vi "836_Safe Image Get Image.vi"(6 "Video Mode":i32, 8 "error in":errorcluster, 9 "Operation":T3(ring), 10 "Image In":T1, 11 "Session In":T2) -> (0 "error out":errorcluster, 1 "Image Data String":string, 2 "Image Out":T1, 3 "Session Out":T2)   [LabVIEW 2015]
uses:
  <vilib>/userdefined/High Color/IMAQdx.ctl
  <vilib>/vision/Image Controls.llb/IMAQ Image.ctl
  <vilib>/vision/driver/IMAQdx.llb/IMAQdx Buffer Number Mode.ctl
  <resource>/objmgr/imaqdx.rc
  <vilib>/vision/driver/NI_Vision_Acquisition_Software.lvlib
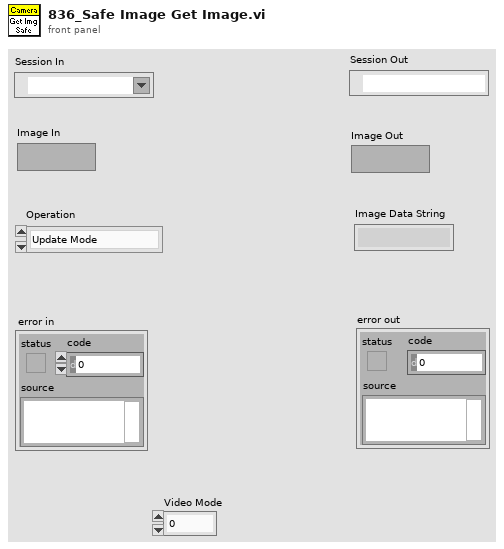
[diagram p1: front panel]
types:
  T1 = typedef "IMAQ Image.ctl" = refnum<image>
  T2 = typedef "IMAQdx.ctl" = refnum<k21>
  T3 = enum16{"Update Mode", "Get Image", "Get Image Data"}
  T4 = typedef "NI_Vision_Acquisition_Software.lvlib/IMAQdx Buffer Number Mode.ctl" = enum32{"Next", "Last", "Buffer Number", "Every", "Last New"}
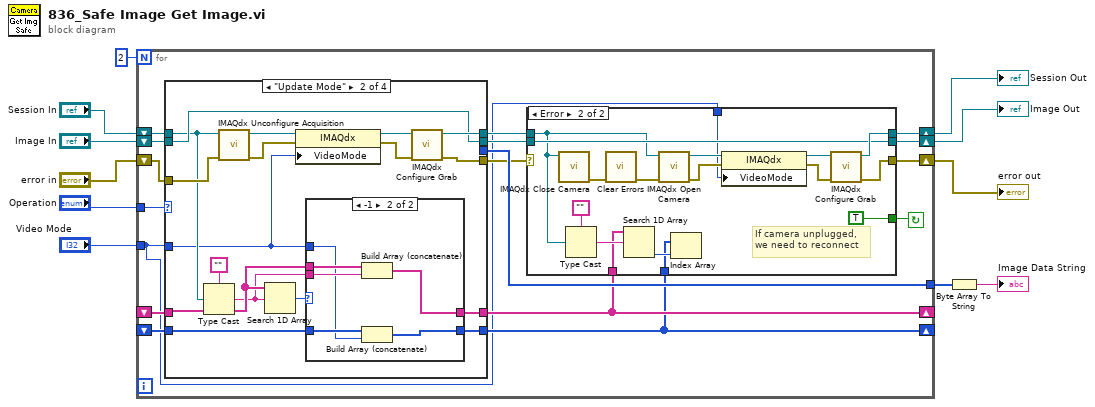
[diagram p0: block diagram]
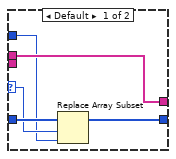
[diagram p4: hidden frame]
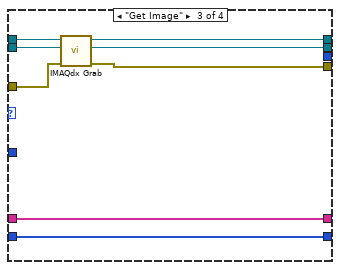
[diagram p5: hidden frame]
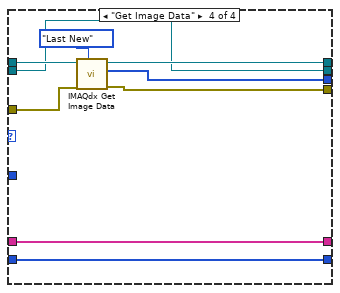
[diagram p6: hidden frame]
diagram:
  n1 = for {
    N: 2 -> [_]
    tunnel: "Operation" -> [w28]
    tunnel: "Video Mode" -> [w12]
    tunnel: [w24] -> w7
    shift-right: [w18] -> w3
    shift-left: "Session In" -> [w27]
    shift-right: [w20] -> w4
    shift-left: "Image In" -> [w26]
    shift-right: [w22] -> w5
    shift-left: "error in" -> [w25]
    shift-right: [w14] -> _
    shift-left: _ -> [w16]
    shift-right: [w13] -> _
    shift-left: _ -> [w15]
    stop <- w17 continue-if-true
    n2 = case shown="\"Update Mode\"" w28 {
      tunnel: w27 -> [w53 w59 w89 w94]
      tunnel: [w53 w68 w86 w96] -> w19
      tunnel: [w52 w66 w84 w95] -> w23
      tunnel: w12 -> [_ w55 _ _]
      tunnel: w26 -> [w51 w63 w88 w92]
      tunnel: [w51 w63 w85 w92] -> w21
      tunnel: [_ _ _ w97] -> w24
      tunnel: w25 -> [w52 w64 w87 w93]
      tunnel: w16 -> [w50 w61 w83 w91]
      tunnel: w15 -> [w49 w60 w82 w90]
      tunnel: [w50 w56 w83 w91] -> w14
      tunnel: [w49 w54 w82 w90] -> w13
      frame Default {
      }
      frame "Update Mode" {
        n3 = Type Cast(type="", x=w59) -> (*(type *) &x=w57:string)
        n4 = call <vilib>:"IMAQdx Unconfigure Acquisition.vi"("error in"=w64, "Session In"=w59) -> ("error out"=w65:errorcluster, "Session Out"=w70:T2)  [unwired: 8 in]
        n5 = Search 1D Array(1D array=w61, element=w57) -> (index of element=w62:i32)  [unwired: 1 in]
        n6 = property class="IMAQdx"(reference=w70, error in=w65, "VideoMode"=w55) -> (reference out=w69:T2, error out=w67:errorcluster)
        n7 = case shown="-1" w62 {
          selector: w62 -> [w73 _]
          tunnel: w61 -> [w75 w81]
          tunnel: w60 -> [w74 w78]
          tunnel: w57 -> [_ w80]
          tunnel: [w75 w79] -> w56
          tunnel: w55 -> [w72 w76]
          tunnel: [w71 w77] -> w54
          frame Default {
            n8 = Replace Array Subset(array=w74, new element=w72, index=w73) -> (w71:i32[])
          }
          frame -1 {
            n9 = Build Array (concatenate)(w81, w80) -> (w79:string[])
            n10 = Build Array (concatenate)(w78, w76) -> (w77:i32[])
          }
        }
        n11 = call <vilib>:"IMAQdx Configure Grab.vi"("error in"=w67, "Session In"=w69) -> ("error out"=w66:errorcluster, "Session Out"=w68:T2)  [unwired: 8 in]
      }
      frame "Get Image" {
        n12 = call <vilib>:"IMAQdx Grab.vi"("error in"=w87, "Image In"=w88, "Session In"=w89) -> ("error out"=w84:errorcluster, "Image Out"=w85:T1, "Session Out"=w86:T2)  [unwired: 5 in, 1 out]
      }
      frame "Get Image Data" {
        n13 = call <vilib>:"IMAQdx Get Image Data.vi"("Buffer Number Mode (Next)"=IMAQdx_Buffer_Number_Mode."Last New", "error in"=w93, "Session In"=w94) -> ("error out"=w95:errorcluster, "Image Data Array"=w97:u8[], "Session Out"=w96:T2)  [unwired: 5 in, 1 out]
      }
    }
    n14 = case shown="Error" w23 {
      selector: w23 -> [w31 _]
      tunnel: [w31 w44] -> w22
      tunnel: w21 -> [w30 w45]
      tunnel: [w30 w45] -> w20
      tunnel: w19 -> [w29 w37]
      tunnel: [w29 w46] -> w18
      tunnel: [_ TRUE] -> w17
      tunnel: w14 -> [_ w35]
      tunnel: w13 -> [_ w33]
      tunnel: w12 -> [_ w32]
      frame No Error {
      }
      frame Error {
        # "If camera unplugged,\nwe need to reconnect"
        n15 = call <vilib>:"IMAQdx Close Camera.vi"("Session In"=w37) -> ("error out"=w48:errorcluster)  [unwired: 10 in]
        n16 = Type Cast(type="", x=w37) -> (*(type *) &x=w36:string)
        n17 = call <vilib>:"Clear Errors.vi"("error in (no error)"=w48) -> ("error out"=w47:errorcluster)  [unwired: 5 in, 1 out]
        n18 = Search 1D Array(1D array=w35, element=w36) -> (index of element=w34:i32)  [unwired: 1 in]
        n19 = call <vilib>:"IMAQdx Open Camera.vi"("error in"=w47, "Session In"=w37) -> ("error out"=w40:errorcluster, "Session Out"=w42:T2)  [unwired: 8 in]
        n20 = Index Array(array=w33, index=w34) -> ()  [unwired: 1 out]
        n21 = property class="IMAQdx"(reference=w42, error in=w40, "VideoMode"=w32) -> (reference out=w41:T2, error out=w39:errorcluster)
        n22 = call <vilib>:"IMAQdx Configure Grab.vi"("error in"=w39, "Session In"=w41) -> ("error out"=w44:errorcluster, "Session Out"=w46:T2)  [unwired: 8 in]
      }
    }
  }
  "Session Out" <- w3
  "Image Out" <- w4
  "error out" <- w5
  n23 = Byte Array To String(unsigned byte array=w7) -> (string=→"Image Data String":string)
